vi "Get Device IDs.vi"(8 "error in (no error)":errorcluster, 9 "Device and Axis":string, 11 "VISA resource name":refnum<visa-resource-name>) -> (0 "error out":errorcluster, 1 "Peripheral ID":i32, 2 "Device ID":i32, 3 "VISA resource name out":refnum<visa-resource-name>)   [LabVIEW 2013, in "Zaber A Series.lvlib"]
doc: "Returns the numeric device ID and peripheral ID if appropriate for one device and optional axis. The outputs can be used with the Look Up Device Properties VI to get information about the device such as its name and microstep size. \n\nThis VI is meant to work with only one device or one device and one axis at a time. Providing a device and axis input that matches multiple devices produces undefined behavior. When addressing a standalone controller, the first axis is assumed unless you specify an axis number or zero to get information about the controller itself.\n\nThis VI requires that the Initialize VI has been called with the same serial port."
uses:
  Zaber A Series.lvlib
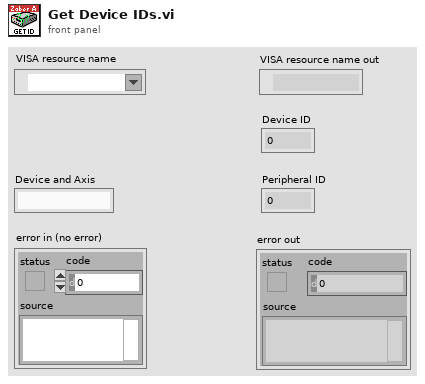
[diagram p1: front panel]
types:
  T1 = cluster{"Device":string, "Axis":string, "Reply Flag":string, "Status":string, "Warning Flags":string, "Data":string}[]
  T2 = cluster{"Device":string, "Axis":string, "Reply Flag":string, "Status":string, "Warning Flags":string, "Data":string}
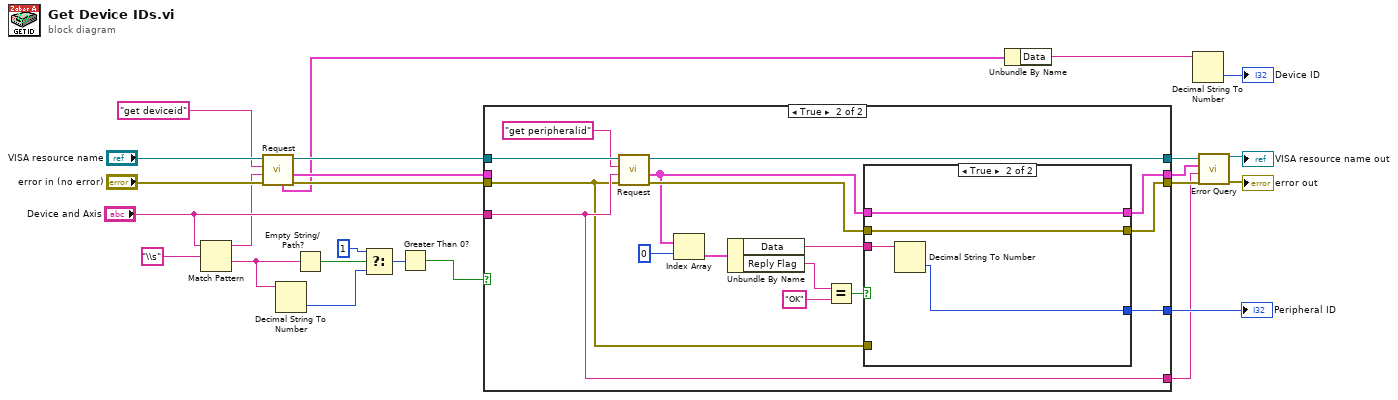
[diagram p0: block diagram]
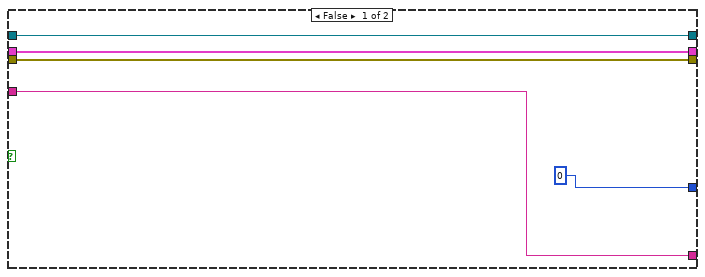
[diagram p2: hidden frame]
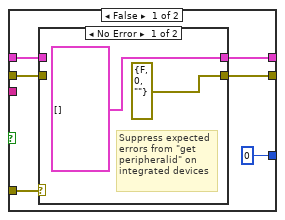
[diagram p3: hidden frame]
diagram:
  n1 = Match Pattern(string="Device and Axis", regular expression="\\s") -> (before substring=w10:string, after substring=w20:string)  [unwired: 1 in, 2 out]
  n2 = call "Request.vi"("error in (no error)"="error in (no error)", "Device and Axis"=w10, "Command String"="get deviceid", "VISA resource name"="VISA resource name") -> ("error out"=w12:errorcluster, "Response Bundle Array"=w4:T1, "VISA resource name out"=w13:refnum<visa-resource-name>, "First Response Bundle"=w1:T2)  [unwired: 2 in, 2 out]
  n3 = Decimal String To Number(string=w20) -> (number=w18:i32)  [unwired: 2 in, 1 out]
  n4 = Empty String/Path?(string/path=w20) -> (empty?=w19:bool)
  n5 = Select(t=1 ("f"), s=w19, f=w18) -> (s? t:f=w16:i32)
  n6 = Greater Than 0?(x=w16) -> (x > 0?=w21:bool)
  n7 = case shown="True" w21 {
    tunnel: w13 -> [w30 w45]
    tunnel: w12 -> [w29 w31]
    tunnel: [w29 w34] -> w8
    tunnel: [0 w46] -> w23
    tunnel: [w30 w44] -> w7
    tunnel: "Device and Axis" -> [w26 w36]
    tunnel: w4 -> [w27 _]
    tunnel: [w27 w32] -> w3
    tunnel: [w26 w36] -> w2
    frame False {
    }
    frame True {
      n8 = call "Request.vi"("error in (no error)"=w31, "Device and Axis"=w36, "Command String"="get peripheralid", "VISA resource name"=w45) -> ("error out"=w35:errorcluster, "Response Bundle Array"=w33:T1, "VISA resource name out"=w44:refnum<visa-resource-name>)  [unwired: 2 in, 3 out]
      n9 = Index Array(array=w33, index=0) -> (element=w38:T2)
      n10 = Unbundle By Name(w38) -> ("Data"=w42:string, "Reply Flag"=w41:string)
      n11 = Equal?(x=w41, y="OK") -> (x = y?=w40:bool)
      n12 = case shown="True" w40 {
        tunnel: w42 -> [_ w60]
        tunnel: [0 w59] -> w46
        tunnel: w35 -> [w50 w58]
        tunnel: [w49 w58] -> w34
        tunnel: w33 -> [w47 w57]
        tunnel: [w48 w57] -> w32
        tunnel: w31 -> [w51 _]
        frame False {
          n13 = case shown="No Error" w51 {
            tunnel: w50 -> [_ w56]
            tunnel: [errorcluster {"status"=FALSE, "code"=0, "source"=""} ("error out") w56] -> w49
            tunnel: [T1 [] ("Response Bundle Array") w55] -> w48
            tunnel: w47 -> [_ w55]
            frame No Error {
              # "Suppress expected\nerrors from \"get\nperipheralid\" on \nintegrated devices"
            }
            frame Error {
            }
          }
        }
        frame True {
          n14 = Decimal String To Number(string=w60) -> (number=w59:i32)  [unwired: 2 in, 1 out]
        }
      }
    }
  }
  "Peripheral ID" <- w23
  n15 = Unbundle By Name(w1) -> ("Data"=w25:string)
  n16 = Decimal String To Number(string=w25) -> (number=→"Device ID":i32)  [unwired: 2 in, 1 out]
  n17 = call "Error Query.vi"("error in (no error)"=w8, "Device and Axis"=w2, "Previous Response Bundle Array"=w3, "VISA resource name"=w7) -> ("error out"=→"error out":errorcluster, "VISA resource name out"=→"VISA resource name out":refnum<visa-resource-name>)  [unwired: 4 in, 2 out]
